vi "GV-LegendMoveAction.vi"(8 "error in (no error)":errorcluster, 9 "Coords":T1, 11 "Gviewer in":refnum<class "Gviewer.lvclass">) -> (0 "error out":errorcluster, 1 "Plot Images:Front":picture, 3 "Gviewer out":refnum<class "Gviewer.lvclass">)   [LabVIEW 2020, in "Sgraph_lib_V1.lvlib" / "Gviewer.lvclass"]
doc: "Andre Koelewijn, 27 April 2021\n\nMove legend over the graph area"
uses:
  Gviewer.lvclass
  <vilib>/Utility/miscctls.llb/LVPoint32TypeDef.ctl
  Gviewer.lvclass/Gviewer.ctl
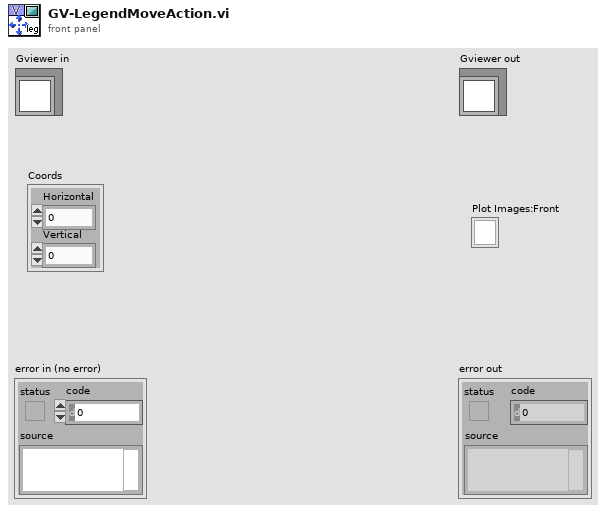
[diagram p1: front panel]
types:
  T1 = typedef "LVPoint32TypeDef.ctl" = cluster{"Horizontal":i32, "Vertical":i32}
  T2 = typedef "LVPositionTypeDef.ctl" = cluster{"Left":i32, "Top":i32}
  T3 = typedef "LVRectTypeDef.ctl" = cluster{"Left":i16, "Top":i16, "Right":i16, "Bottom":i16}
  T4 = typedef "LVBoundsTypeDef.ctl" = cluster{"Width":u32, "Height":u32}
  T5 = typedef "Sgraph_lib_V1.lvlib/Gviewer.lvclass/LegendSet.ctl" = cluster{"Position":T2, "Size":T4, "Rows":u32, "Select":i32, "Visible":bool}
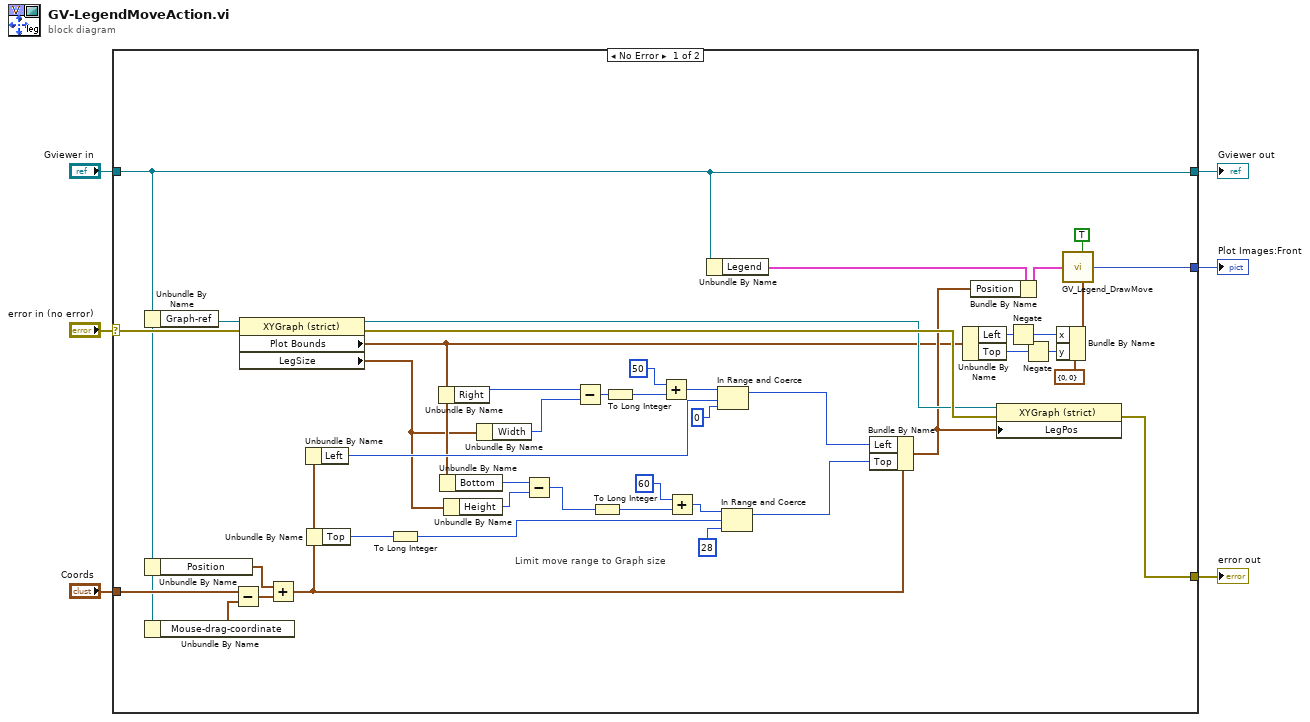
[diagram p0: block diagram]
diagram:
  n1 = case shown="No Error" "error in (no error)" {
    selector: "error in (no error)" -> [w35 w51]
    tunnel: [w32 w51] -> w5
    tunnel: [w30 w50] -> w3
    tunnel: "Gviewer in" -> [w30 w50]
    tunnel: "Coords" -> [w34 _]
    tunnel: [w33 _] -> w1
    frame No Error {
      # "Limit move range to Graph size"
      n2 = Unbundle By Name(w30) -> ("Graph-ref"=w38:refnum<vi>)
      n3 = Unbundle By Name(w30) -> ("Position"=w48:T2)
      n4 = Unbundle By Name(w30) -> ("Mouse-drag-coordinate"=w49:T1)
      n5 = Subtract(x=w34, y=w49) -> (x-y=w47:T1)
      n6 = property class="XYGraph (strict)"(reference=w38, error in=w35) -> (reference out=w31:refnum<vi>, error out=w39:errorcluster, "Plot Bounds"=w15:T3, "LegSize"=w12:T4)
      n7 = Add(x=w48, y=w47) -> (x+y=w19:T2)
      n8 = Unbundle By Name(w19) -> ("Left"=w26:i32)
      n9 = Unbundle By Name(w19) -> ("Top"=w17:i32)
      n10 = To Long Integer(number=w17) -> (32bit integer=w8:i32)
      n11 = Unbundle By Name(w15) -> ("Right"=w24:i16)
      n12 = Unbundle By Name(w15) -> ("Bottom"=w14:i16)
      n13 = Unbundle By Name(w12) -> ("Height"=w13:u32)
      n14 = Unbundle By Name(w12) -> ("Width"=w27:u32)
      n15 = Subtract(x=w14, y=w13) -> (x-y=w10:u32)
      n16 = Subtract(x=w24, y=w27) -> (x-y=w23:u32)
      n17 = To Long Integer(number=w10) -> (32bit integer=w7:i32)
      n18 = To Long Integer(number=w23) -> (32bit integer=w22:i32)
      n19 = Add(x=50, y=w22) -> (x+y=w20:i32)
      n20 = Add(x=60, y=w7) -> (x+y=w9:i32)
      n21 = Unbundle By Name(w30) -> ("Legend"=w37:T5)
      n22 = In Range and Coerce(upper limit=w20, x=w26, lower limit=0) -> (coerced(x)=w28:i32)  [unwired: 1 out]
      n23 = In Range and Coerce(upper limit=w9, x=w8, lower limit=28) -> (coerced(x)=w18:i32)  [unwired: 1 out]
      n24 = Bundle By Name(cluster=w19, "Left"=w28, "Top"=w18) -> (w29:T2)
      n25 = Unbundle By Name(w15) -> ("Left"=w42:i16, "Top"=w44:i16)
      n26 = Bundle By Name(cluster=w37, "Position"=w29) -> (w36:T5)
      n27 = property class="XYGraph (strict)"(reference=w31, error in=w39, "LegPos"=w29) -> (error out=w32:errorcluster)  [unwired: 1 out]
      n28 = Negate(x=w42) -> (-x=w43:i16)
      n29 = Negate(x=w44) -> (-x=w45:i16)
      n30 = Bundle By Name(cluster=cluster{"x":i16, "y":i16} {"x"=0, "y"=0}, "x"=w43, "y"=w45) -> (w40:cluster{"x":i16, "y":i16})
      n31 = call "GV_Legend_DrawMove.vi"("Legend"=w36, "Select"=TRUE, "Origin"=w40) -> ("Image"=w33:picture)  [unwired: 6 in]
    }
    frame Error {
    }
  }
  "error out" <- w5
  "Gviewer out" <- w3
  "Plot Images:Front" <- w1
